vi "startClockwise.vi"   [LabVIEW 2012]
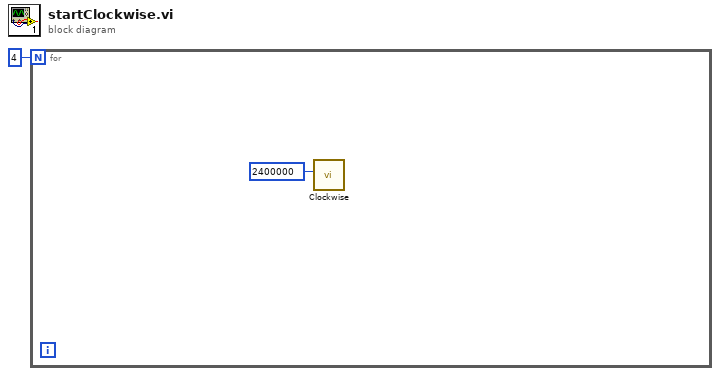
[diagram p0: block diagram]
diagram:
  n1 = for {
    N: 4 -> [_]
    n2 = call "Clockwise.vi"("Count(Ticks)"=u32 2400000) -> ()  [unwired: 11 in]
  }
